vi "题目3.vi"() -> ()   [LabVIEW 2017]
panel:
  out "温度":string
  in  "温度单位":bool
  in  "停止":bool
  out "温度计":dbl(slide) scale=0.0..100.0
  # "°F"
  # "°C"
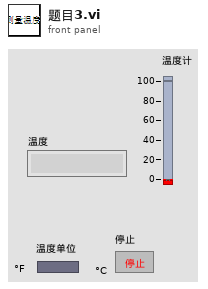
[diagram p1: front panel]
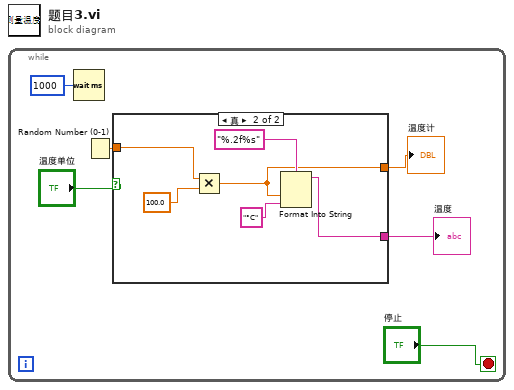
[diagram p0: block diagram]
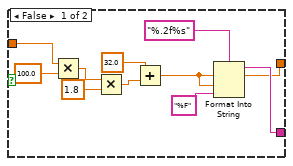
[diagram p2: hidden frame]
diagram:
  n1 = while {
    stop <- "停止" stop-if-true
    n2 = Wait (ms)(milliseconds to wait=u32 1000 ("等待时间（毫秒）")) -> ()  [unwired: 1 out]
    n3 = Random Number (0-1)() -> (number: 0 to 1=w5:dbl)
    n4 = case shown="真" "温度单位" {
      tunnel: w5 -> [w16 w21]
      tunnel: [w7 w18] -> w4
      tunnel: [w8 w17] -> w3
      frame False {
        n5 = Multiply(x=w16, y=100.0) -> (x*y=w14:dbl)
        n6 = Multiply(x=w14, y=1.8) -> (x*y=w12:dbl)
        n7 = Add(x=32.0, y=w12) -> (x+y=w7:dbl)
        n8 = Format Into String(format string="%.2f%s" ("格式字符串"), w7, "%F") -> (resulting string=w8:string)  [unwired: 2 in, 1 out]
      }
      frame True {
        n9 = Multiply(x=w21, y=100.0) -> (x*y=w18:dbl)
        n10 = Format Into String(format string="%.2f%s" ("格式字符串"), w18, "°C") -> (resulting string=w17:string)  [unwired: 2 in, 1 out]
      }
    }
    "温度计" <- w4
    "温度" <- w3
  }
